vi "InsertClonedHierarchy.vi"(8 "error in (no error)":errorcluster, 9 "Root path":path, 10 "Dependency List in":refnum<class "CDependencyList.lvclass">, 11 "CDependencyList in":refnum<class "CDependencyList.lvclass">) -> (0 "error out":errorcluster, 3 "CDependencyList out":refnum<class "CDependencyList.lvclass">)   [LabVIEW 2020, in "DependencyInspection.lvlib" / "CDependencyList.lvclass"]
uses:
  CDependencyList.lvclass
  obj/Addons/LabVIEWObjectInterfaces.lvlibp/LabVIEWObjectInterfaces/ILabVIEWItem/ILabVIEWItem.lvclass
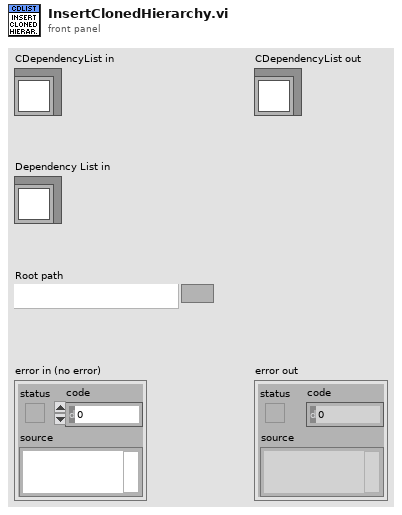
[diagram p1: front panel]
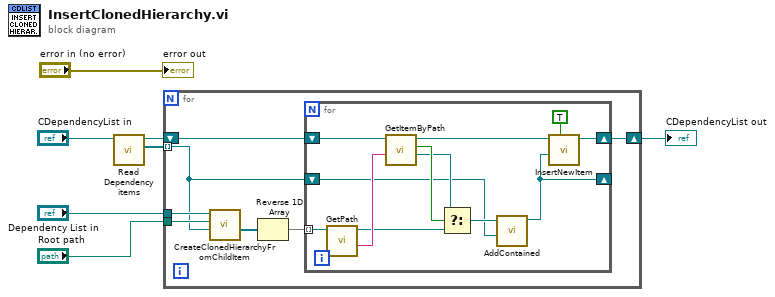
[diagram p0: block diagram]
diagram:
  n1 = call-dynamic "Read Dependency items.vi"("CDependencyList in"="CDependencyList in") -> ("Dependency items"=w1:refnum<class "ILabVIEWItem.lvclass">[], "CDependencyList out"=w2:refnum<class "CDependencyList.lvclass">)  [unwired: 9 in]
  n2 = for {
    tunnel: "Dependency List in" -> [w12]
    tunnel: "Root path" -> [w11]
    shift-right: [w9] -> w4
    shift-left: w2 -> [w10]
    tunnel: w1 -> [w8] mode=indexing
    n3 = call-dynamic "CreateClonedHierarchyFromChildItem.vi"("ILabVIEWItem to clone"=w8, "Root path"=w11, "CDependencyList in"=w12) -> ("Hierarchy items"=w14:refnum<class "ILabVIEWItem.lvclass">[])  [unwired: 6 in, 2 out]
    n4 = Reverse 1D Array(array=w14) -> (reversed array=w13:refnum<class "ILabVIEWItem.lvclass">[])
    n5 = for {
      tunnel: w13 -> [w25] mode=indexing
      shift-right: [w17] -> w9
      shift-left: w10 -> [w26]
      shift-right: [w16] -> _
      shift-left: w8 -> [w15]
      n6 = call-dynamic "GetPath.vi"("ILabVIEWItem in"=w25) -> ("Path"=w24:string, "ILabVIEWItem out"=w21:refnum<class "ILabVIEWItem.lvclass">)  [unwired: 8 in, 1 out]
      n7 = call-dynamic "GetItemByPath.vi"("Path"=w24, "CDependencyList in"=w26) -> ("ILabVIEWItem"=w22:refnum<class "ILabVIEWItem.lvclass">, "key found?"=w23:bool, "CDependencyList out"=w18:refnum<class "CDependencyList.lvclass">)  [unwired: 6 in, 1 out]
      n8 = Select(t=w22, s=w23, f=w21) -> (s? t:f=w19:refnum<class "ILabVIEWItem.lvclass">)
      n9 = call-dynamic "AddContained.vi"("Item to contain"=w15, "ILabVIEWItem in"=w19) -> ("ILabVIEWItem out"=w16:refnum<class "ILabVIEWItem.lvclass">)  [unwired: 8 in, 1 out]
      n10 = call-dynamic "InsertNewItem.vi"("Replace?"=TRUE, "ILabVIEWItem in"=w16, "CDependencyList in"=w18) -> ("CDependencyList out"=w17:refnum<class "CDependencyList.lvclass">)  [unwired: 6 in, 2 out]
    }
  }
  "CDependencyList out" <- w4
  "error out" <- "error in (no error)"
